vi "Read txt Color.vi"(8 "error in (no error)":errorcluster, 11 "Color Message in":refnum<class "Color Message.lvclass">) -> (0 "error out":errorcluster, 2 "txt Color":u32(colorbox), 3 "Color Message out":refnum<class "Color Message.lvclass">)   [LabVIEW 2020, in "Color Message.lvclass"]
uses:
  Color Message.lvclass
  Color Message.lvclass/Color Message.ctl
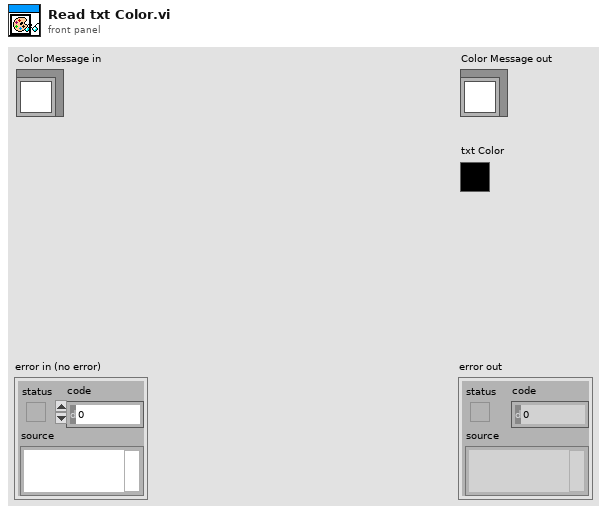
[diagram p1: front panel]
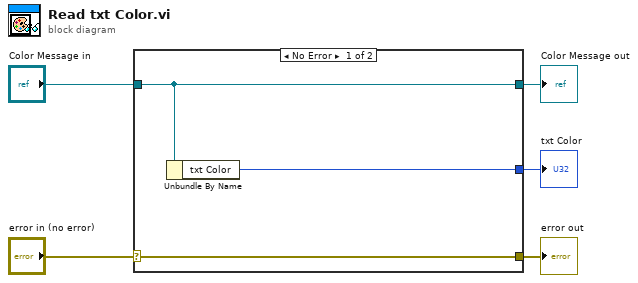
[diagram p0: block diagram]
diagram:
  n1 = case shown="No Error" "error in (no error)" {
    selector: "error in (no error)" -> [w8 w9]
    tunnel: [w8 w9] -> w4
    tunnel: [w7 w10] -> w2
    tunnel: "Color Message in" -> [w7 w10]
    tunnel: [w6 _] -> w1
    frame No Error {
      n2 = Unbundle By Name(w7) -> ("txt Color"=w6:u32)
    }
    frame Error {
    }
  }
  "error out" <- w4
  "Color Message out" <- w2
  "txt Color" <- w1
